vi "Teleop.vi"(10 "Match Info":T1={"Autonomous Elapsed Seconds"=0.0, "TeleOp Elapsed Seconds"=0.0, "Disabled Elapsed Seconds"=0.0, "Visited Autonomous"=FALSE, "Visited TeleOp"=FALSE, "Visited Disabled"=FALSE, "Autonomous Settings"={"Autonomous Style"=enum."Independent", "VI Refnum"=refnum}}, 11 "Call Context":T2) -> ()   [LabVIEW 2012]
doc: "This VI is called for each TeleOp packet received from the DS where the robot is not disabled. It is often used to read from the joysticks and update I/O or to update setpoints for timed control loops. It should complete and return within 20 milliseconds or it may miss DS packets."
uses:
  <vilib>/Rock Robotics/WPI/DriverStation/WPI_DriverStationDerivedRobotMode.ctl
  <vilib>/Rock Robotics/WPI/DriverStation/WPI_DriverStationMatch Info.ctl
  Robot Global Data.vi
  <vilib>/Rock Robotics/WPI/Solenoid/Deprecated/WPI_SolenoidSetBool.vi
  <vilib>/Rock Robotics/WPI/Joystick/WPI_JoystickGetSetRefNum.vi
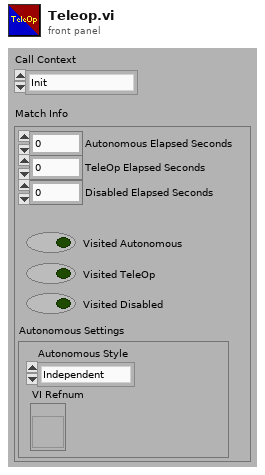
[diagram p1: front panel]
types:
  T1 = typedef "WPI_DriverStationMatch Info.ctl" = cluster{"Autonomous Elapsed Seconds":dbl, "TeleOp Elapsed Seconds":dbl, "Disabled Elapsed Seconds":dbl, "Visited Autonomous":bool, "Visited TeleOp":bool, "Visited Disabled":bool, "Autonomous Settings":cluster{"Autonomous Style":enum16{"Iterative", "Independent"}, "VI Refnum":refnum<vi>}}
  T2 = typedef "WPI_DriverStationDerivedRobotMode.ctl" = enum16{"Init", "Execute", "Stop"}
  T3 = typedef "WPI_DigitalInputDevRef.ctl" = cluster{"DevStatus":errorcluster, "DIO Channel":T4, "Digital Module":T5}
  T4 = typedef "FPGA_DIOChannel.ctl" = enum8{"DIO 1", "DIO 2", "DIO 3", "DIO 4", "DIO 5", "DIO 6", "DIO 7", "DIO 8", "DIO 9", "DIO 10", "DIO 11", "DIO 12", "DIO 13", "DIO 14", "Invalid"}
  T5 = typedef "FPGA_TypedefDigitalModule.ctl" = enum16{"Digital Module 1", "Digital Module 2"}
  T6 = typedef "WPI_MotorControlDeviceRef.ctl" = cluster{"DeviceStatus":errorcluster, "Type":enum16{"PWM", "CAN"}, "PWM":cluster{"Digital Module":T5, "PWM Channel":T7, "DeadBand":T8}, "CAN":cluster{"Device Number":u8, "Control Mode":T9, "Semaphore":T10, "Max Vout":dbl}, "Invert":bool, "TransformRef":T11, "InvTransformRef":T11}
  T7 = typedef "FPGA_DIOPWMChannel.ctl" = enum8{"PWM 1", "PWM 2", "PWM 3", "PWM 4", "PWM 5", "PWM 6", "PWM 7", "PWM 8", "PWM 9", "PWM 10", "Invalid"}
  T8 = typedef "WPI_PWMDeadband.ctl" = cluster{"Name":string, "maxPositivePwm":i32, "minPositivePwm":i32, "centerPwm":i32, "maxNegativePwm":i32, "minNegativePwm":i32, "angularRange":u16}
  T9 = typedef "WPI_CANJaguar_ControlMode.ctl" = enum8{"Percent VBus", "Current", "Speed", "Position", "Voltage"}
  T10 = typedef "Semaphore RefNum" = refnum<k1>
  T11 = typedef "WPI_PWMTransform_ConPane.ctl" = refnum<vi>
  T12 = typedef "WPI_JoystickDevRef.ctl" = cluster{"Device":T13}
  T13 = typedef "WPI_JoystickDeviceEnum.ctl" = enum16{"USB 1", "USB 2", "USB 3", "USB 4", "Kinect 1", "Kinect 2"}
  T14 = typedef "WPI_SolenoidDevRef.ctl" = cluster{"DevStatus":errorcluster, "Solenoid Module":T15, "Forward Solenoid Channel":T16, "Reverse Solenoid Channel":T16}
  T15 = typedef "FPGA_TypedefSolenoidModule.ctl" = enum16{"Solenoid Module 1", "Solenoid Module 2"}
  T16 = typedef "WPI_SolenoidChannel.ctl" = enum8{"Solenoid 1", "Solenoid 2", "Solenoid 3", "Solenoid 4", "Solenoid 5", "Solenoid 6", "Solenoid 7", "Solenoid 8", "Invalid"}
  T17 = typedef "WPI_JoystickButtonState.ctl" = cluster{"Button 1":bool, "Button 2":bool, "Button 3":bool, "Button 4":bool, "Button 5":bool, "Button 6":bool, "Button 7":bool, "Button 8":bool, "Button 9":bool, "Button 10":bool, "Button 11":bool, "Button 12":bool}
  T18 = cluster{"axis 1 (x)":dbl, "axis 2 (y)":dbl, "axis 3 (throttle)":dbl, "axis 4":dbl, "axis 5":dbl, "axis 6":dbl}
  T19 = typedef "WPI_RobotDriveDevRef.ctl" = cluster{"DevStatus":errorcluster, "Motors[]":T6[], "Square Inputs":bool, "Max Output":dbl, "Isochronous":bool}
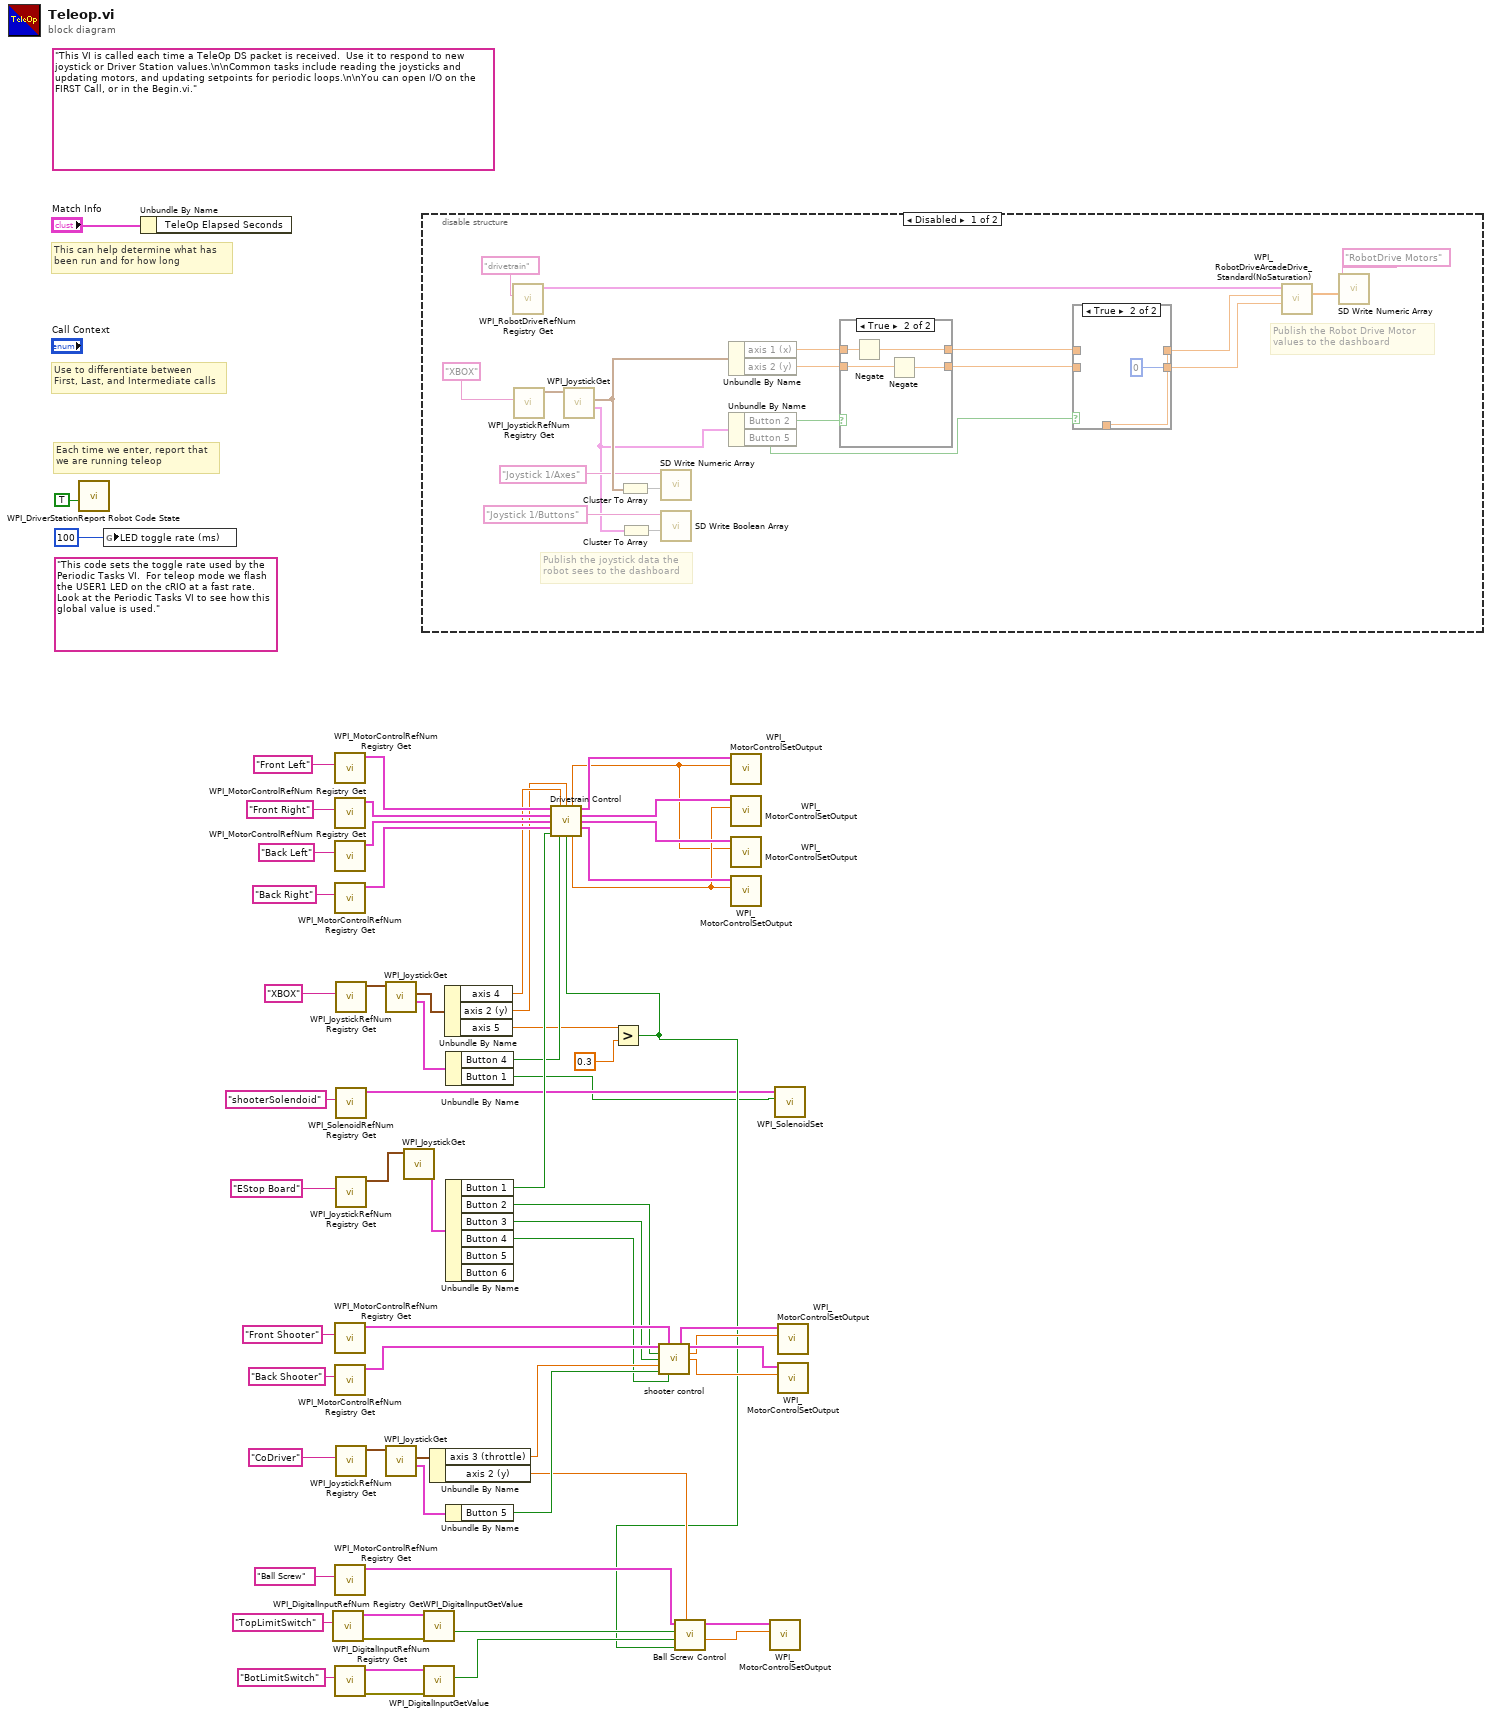
[diagram p0: block diagram]
diagram:
  (unwired) "This code sets the toggle rate used by the Periodic Tasks VI.  For teleop mode we flash the USER1 LED on the cRIO at a fast rate.  Look at the Periodic Tasks VI to see how this global value is used."
  (unwired) "This VI is called each time a TeleOp DS packet is received.  Use it to respond to new joystick or Driver Station values.\n\nCommon tasks include reading the joysticks and updating motors, and updating setpoints for periodic loops.\n\nYou can open I/O on the FIRST Call, or in the Begin.vi."
  # "Each time we enter, report that\nwe are running teleop"
  # "Use to differentiate between\nFirst, Last, and Intermediate calls"
  # "This can help determine what has\nbeen run and for how long"
  n1 = call <vilib>:"WPI_DriverStationReport Robot Code State.vi"("TeleOp"=TRUE ("Autonomous")) -> ()  [unwired: 10 in, 1 out]
  n2 = global write "Robot Global Data.vi" "LED toggle rate (ms)"(u32 100 ("LED ms toggle rate")) -> ()
  n3 = Unbundle By Name("Match Info") -> ()  [unwired: 1 out]
  n4 = call <vilib>:"WPI_DigitalInputRefNum Registry Get.vi"("refnum name"="TopLimitSwitch") -> ("error out"=w16:errorcluster, "DigitalInputDevRef"=w15:T3)  [unwired: 9 in]
  n5 = call <vilib>:"WPI_MotorControlRefNum Registry Get.vi"("refnum name"="Front Left") -> ("MotorControlDevRef"=w54:T6)  [unwired: 9 in, 1 out]
  n6 = call <vilib>:"WPI_MotorControlRefNum Registry Get.vi"("refnum name"="Front Right") -> ("MotorControlDevRef"=w53:T6)  [unwired: 9 in, 1 out]
  n7 = call <vilib>:"WPI_MotorControlRefNum Registry Get.vi"("refnum name"="Back Left") -> ("MotorControlDevRef"=w52:T6)  [unwired: 9 in, 1 out]
  n8 = call <vilib>:"WPI_MotorControlRefNum Registry Get.vi"("refnum name"="Back Right") -> ("MotorControlDevRef"=w51:T6)  [unwired: 9 in, 1 out]
  n9 = call <vilib>:"WPI_MotorControlRefNum Registry Get.vi"("refnum name"="Front Shooter") -> ("MotorControlDevRef"=w29:T6)  [unwired: 9 in, 1 out]
  n10 = call <vilib>:"WPI_MotorControlRefNum Registry Get.vi"("refnum name"="Back Shooter") -> ("MotorControlDevRef"=w30:T6)  [unwired: 9 in, 1 out]
  n11 = call <vilib>:"WPI_MotorControlRefNum Registry Get.vi"("refnum name"="Ball Screw") -> ("MotorControlDevRef"=w12:T6)  [unwired: 9 in, 1 out]
  n12 = call <vilib>:"WPI_DigitalInputRefNum Registry Get.vi"("refnum name"="BotLimitSwitch") -> ("error out"=w14:errorcluster, "DigitalInputDevRef"=w13:T3)  [unwired: 9 in]
  n13 = call <vilib>:"WPI_JoystickRefNum Registry Get.vi"("refnum name"="XBOX") -> ("JoystickDevRef"=w49:T12)  [unwired: 1 in, 9 out]
  n14 = call <vilib>:"WPI_SolenoidRefNum Registry Get.vi"("refnum name"="shooterSolendoid") -> ("SolenoidDevRef"=w2:T14)  [unwired: 9 in, 1 out]
  n15 = call <vilib>:"WPI_JoystickRefNum Registry Get.vi"("refnum name"="EStop Board") -> ("JoystickDevRef"=w39:T12)  [unwired: 1 in, 9 out]
  n16 = call <vilib>:"WPI_JoystickRefNum Registry Get.vi"("refnum name"="CoDriver") -> ("JoystickDevRef"=w43:T12)  [unwired: 1 in, 9 out]
  n17 = call <vilib>:"WPI_JoystickGet.vi"("JoystickDevRef"=w49) -> ("Buttons"=w45:T17, "Axes"=w48:T18)  [unwired: 1 in, 4 out]
  n18 = call <vilib>:"WPI_JoystickGet.vi"("JoystickDevRef"=w43) -> ("Buttons"=w41:T17, "Axes"=w42:T18)  [unwired: 1 in, 4 out]
  n19 = call <vilib>:"WPI_JoystickGet.vi"("JoystickDevRef"=w39) -> ("Buttons"=w38:T17)  [unwired: 1 in, 5 out]
  n20 = disable-structure shown="Disabled" {
    frame Disabled {
      # "Publish the Robot Drive Motor\nvalues to the dashboard"
      # "Publish the joystick data the\nrobot sees to the dashboard"
      n21 = call <vilib>:"WPI_RobotDriveRefNum Registry Get.vi"("refnum name"="drivetrain") -> ("RobotDriveDevRef"=w84:T19)  [unwired: 1 in, 9 out]
      n22 = call <vilib>:"WPI_JoystickRefNum Registry Get.vi"("refnum name"="XBOX") -> ("JoystickDevRef"=w82:T12)  [unwired: 1 in, 9 out]
      n23 = call <vilib>:"WPI_JoystickGet.vi"("JoystickDevRef"=w82) -> ("Buttons"=w74:T17, "Axes"=w79:T18)  [unwired: 1 in, 4 out]
      n24 = Cluster To Array(cluster=w79) -> (array=w78:dbl[])
      n25 = Cluster To Array(cluster=w74) -> (array=w81:bool[])
      n26 = call <vilib>:"SD Write Numeric Array.vi"("Numeric Array"=w78, "Name"="Joystick 1/Axes") -> ()  [unwired: 8 in, 2 out]
      n27 = call <vilib>:"SD Write Boolean Array.vi"("Boolean Array"=w81, "Name"="Joystick 1/Buttons") -> ()  [unwired: 8 in, 2 out]
      n28 = Unbundle By Name(w79) -> ("axis 1 (x)"=w72:dbl, "axis 2 (y)"=w71:dbl)
      n29 = Unbundle By Name(w74) -> ("Button 2"=w73:bool, "Button 5"=w70:bool)
      n30 = case shown="True" w73 {
        tunnel: [w91 w92] -> w68
        tunnel: w72 -> [w91 w95]
        tunnel: [w90 w93] -> w66
        tunnel: w71 -> [w90 w94]
        frame False {
        }
        frame True {
          n31 = Negate(x=w95) -> (-x=w92:dbl)
          n32 = Negate(x=w94) -> (-x=w93:dbl)
        }
      }
      n33 = case shown="True" w70 {
        tunnel: [w87 w88] -> w69
        tunnel: w68 -> [w87 _]
        tunnel: [w86 0] -> w67
        tunnel: w66 -> [w86 _]
        tunnel: [_ w88] -> w65
        frame False {
        }
        frame True {
        }
      }
      n34 = call <vilib>:"WPI_RobotDriveArcadeDrive_Standard(NoSaturation).vi"("Y axis value"=w67, "X axis value"=w69, "RobotDriveDevRef"=w84) -> ("Motor Values"=w75:dbl[])  [unwired: 1 in, 7 out]
      n35 = call <vilib>:"SD Write Numeric Array.vi"("Numeric Array"=w75, "Name"="RobotDrive Motors") -> ()  [unwired: 8 in, 2 out]
    }
    frame Enabled {
    }
  }
  n36 = call <vilib>:"WPI_DigitalInputGetValue.vi"("error in (no error)"=w16, "DigitalInputDevRef"=w15) -> ("Value"=w11:bool)  [unwired: 7 in, 2 out]
  n37 = call <vilib>:"WPI_DigitalInputGetValue.vi"("error in (no error)"=w14, "DigitalInputDevRef"=w13) -> ("Value"=w10:bool)  [unwired: 7 in, 2 out]
  n38 = Unbundle By Name(w42) -> ("axis 3 (throttle)"=w23:dbl, "axis 2 (y)"=w9:dbl)
  n39 = Unbundle By Name(w48) -> ("axis 4"=w47:dbl, "axis 2 (y)"=w46:dbl, "axis 5"=w7:dbl)
  n40 = Unbundle By Name(w45) -> ("Button 4"=w19:bool, "Button 1"=w1:bool)
  n41 = Unbundle By Name(w38) -> ("Button 1"=w31:bool, "Button 2"=w22:bool, "Button 3"=w21:bool, "Button 4"=w20:bool)  [unwired: 2 out]
  n42 = Unbundle By Name(w41) -> ("Button 5"=w24:bool)
  n43 = Greater?(x=w7, y=0.3) -> (0:w6:bool)
  n44 = call "Drivetrain Control.vi"("Back Left DevRef In"=w54, "X Axis"=w47, "Y Axis"=w46, "Back Right DevRef In"=w53, "Front Left DevRef In"=w52, "Front Right DevRef In"=w51, "Closed Loop On/Off"=w31, "Drivetrain Reverse Button"=w19, "triggerAxis"=w6) -> ("Left Motor Value"=w32:dbl, "Back Left DevRef Out"=w37:T6, "Back Right DevRef Out"=w36:T6, "Front Left DevRef Out"=w35:T6, "Front Right DevRef Out"=w34:T6, "Right Motor Value"=w33:dbl)  [unwired: 1 in]
  n45 = call "shooter control.vi"("Back Shooter DevRef In"=w30, "Front Shooter DevRef In"=w29, "Closed Loop On/Off"=w22, "Power On/Off"=w21, "Joystick Throttle"=w23, "Target Button"=w24, "PyramidButton"=w20) -> ("Front Shooter DevRef Out"=w28:T6, "Back Shooter DevRef Out"=w27:T6, "FrontShooterOut"=w26:dbl, "BackShooterOut"=w25:dbl)  [unwired: 5 in]
  n46 = call "Ball Screw Control.vi"("currentAxis"=w9, "Closed Loop On/Off"=w6, "bottomLimitSwitch"=w10, "topLimitSwitch"=w11, "Ball Screw DevRef In"=w12) -> ("MotorOutput"=w4:dbl, "MotorDevRefOut"=w5:T6)  [unwired: 5 in]
  n47 = call <vilib>:"WPI_MotorControlSetOutput.vi"("Output"=w32, "MotorControlDevRef"=w37) -> ()  [unwired: 7 in, 3 out]
  n48 = call <vilib>:"WPI_MotorControlSetOutput.vi"("Output"=w33, "MotorControlDevRef"=w36) -> ()  [unwired: 7 in, 3 out]
  n49 = call <vilib>:"WPI_MotorControlSetOutput.vi"("Output"=w32, "MotorControlDevRef"=w35) -> ()  [unwired: 7 in, 3 out]
  n50 = call <vilib>:"WPI_MotorControlSetOutput.vi"("Output"=w33, "MotorControlDevRef"=w34) -> ()  [unwired: 7 in, 3 out]
  n51 = call <vilib>:"WPI_MotorControlSetOutput.vi"("Output"=w4, "MotorControlDevRef"=w5) -> ()  [unwired: 7 in, 3 out]
  n52 = call-poly <vilib>:"WPI_SolenoidSet.vi"("Value"=w1, "SolenoidDevRef"=w2) -> ()  [unwired: 8 in, 2 out]
  n53 = call <vilib>:"WPI_MotorControlSetOutput.vi"("Output"=w26, "MotorControlDevRef"=w28) -> ()  [unwired: 7 in, 3 out]
  n54 = call <vilib>:"WPI_MotorControlSetOutput.vi"("Output"=w25, "MotorControlDevRef"=w27) -> ()  [unwired: 7 in, 3 out]
